vi "WaterLevelDetector.vi"() -> ()   [LabVIEW 2019]
panel:
  in  "stop":bool
  out "LED for Lower Level":bool
  out "LED for Upper Level":bool
  in  "Slide":dbl(slide) scale=0.0..10.0
  out "Tank":dbl(slide) scale=0.0..10.0
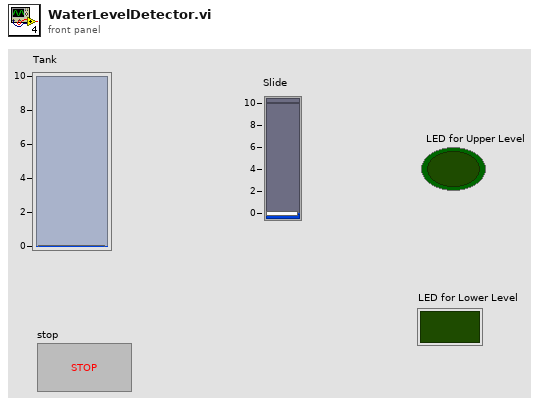
[diagram p1: front panel]
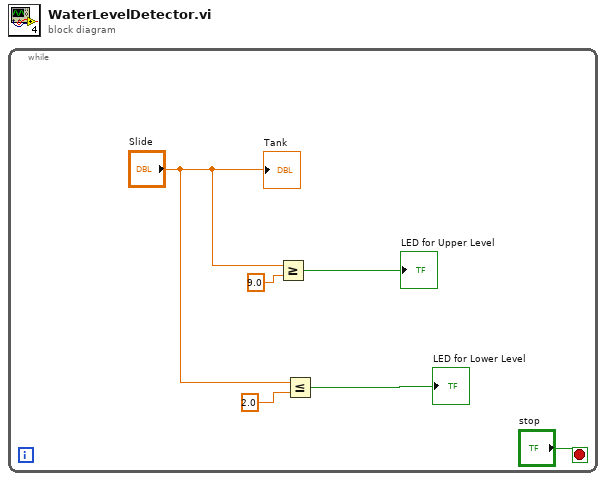
[diagram p0: block diagram]
diagram:
  n1 = while {
    stop <- "stop" stop-if-true
    n2 = Greater Or Equal?(x="Slide", y=9.0) -> (x >= y?=→"LED for Upper Level":bool)
    n3 = Less Or Equal?(x="Slide", y=2.0) -> (x <= y?=→"LED for Lower Level":bool)
    "Tank" <- "Slide"
  }
